vi "RMX41xx Status Check.vi"() -> ()   [LabVIEW 2023]
panel:
  out "Error Code":i32[](array[numeric])
  out "error out":errorcluster
  out "Voltage Output":dbl
  out "Current Output":dbl
  in  "Wait Before Query (1550 ms)":u32=1550
  in  "Output Current (0 A)":dbl
  in  "Output Voltage (0 V)":dbl
  in  "Operation Mode (0: Constant Current)":i32(ring) items=["Constant Current", "Constant Voltage"]
  out "error out 2":errorcluster
  out "Error":bool
  out "Status":i32
  out "resulting string":string
  in  "VISA resource name":refnum<visa-resource-name>="TCPIP0::169.254.100.192::inst0::INSTR"
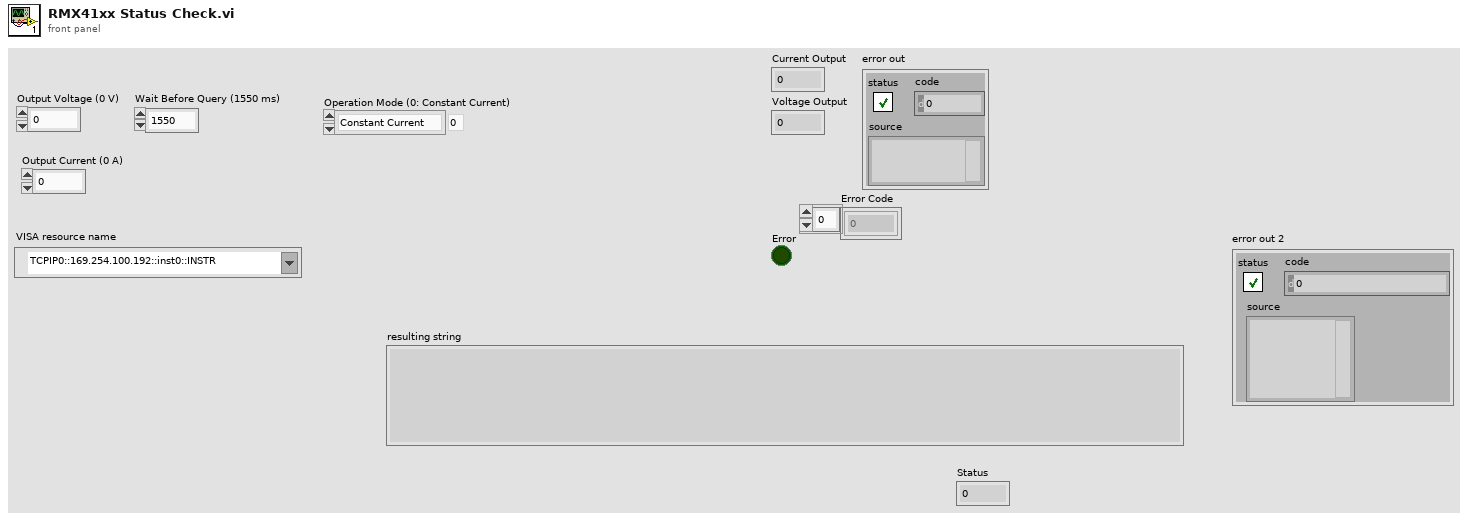
[diagram p1: front panel]
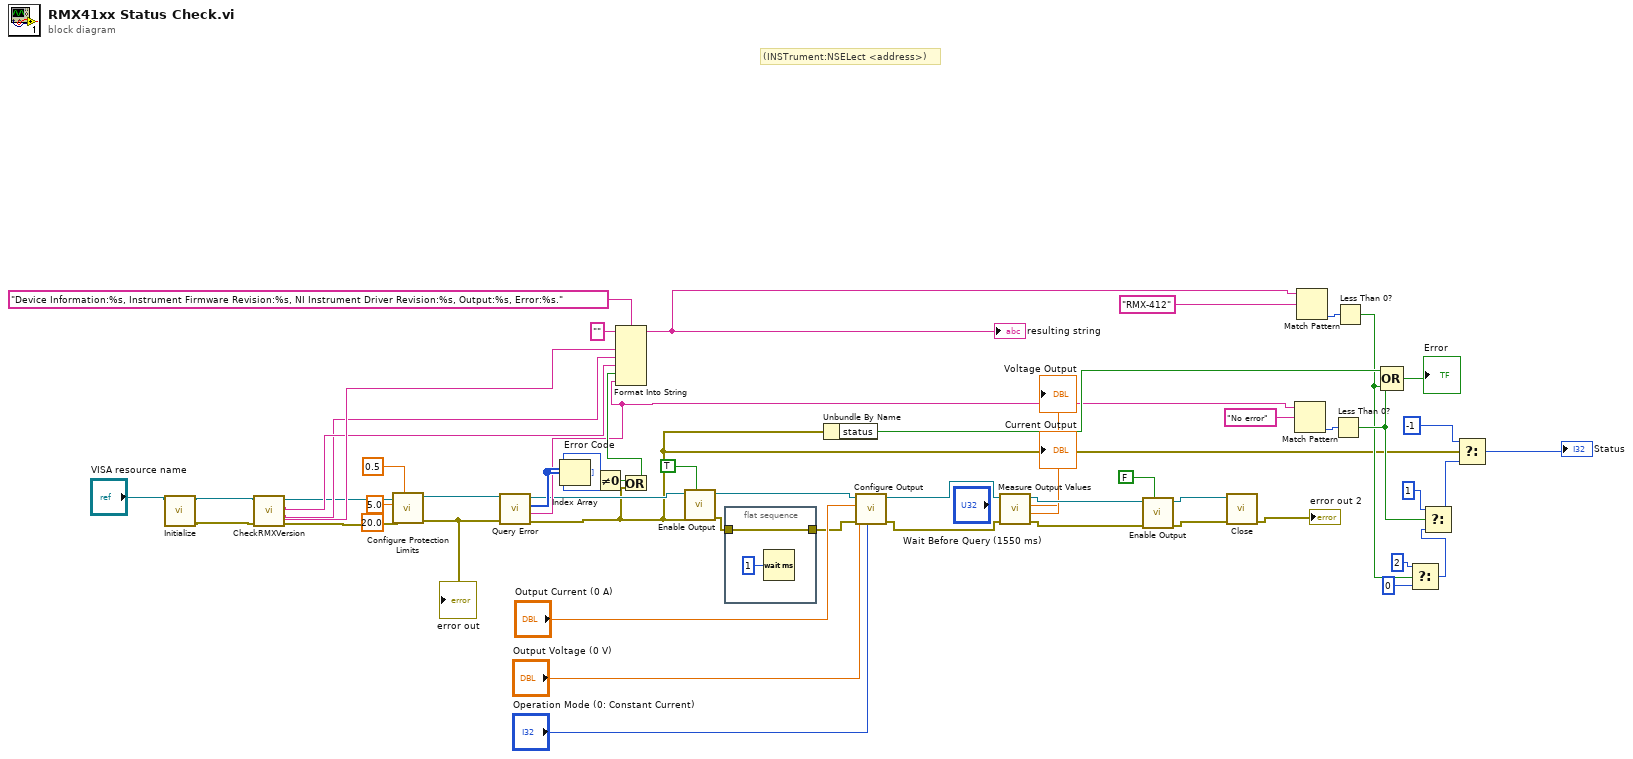
[diagram p0: block diagram]
diagram:
  # "(INSTrument:NSELect <address>)"
  n1 = call "Initialize.vi"("VISA resource name"="VISA resource name") -> ("error out"=w29:errorcluster, "VISA resource name out"=w30:refnum<visa-resource-name>)  [unwired: 9 in]
  n2 = call "CheckRMXVersion.vi"("error in (no error)"=w29, "VISA resource name"=w30) -> ("error out"=w5:errorcluster, "Instrument Driver Revision"=w51:string, "Instrument Firmware Revision"=w52:string, "VISA resource name out"=w7:refnum<visa-resource-name>, "RMXInformation"=w53:string)  [unwired: 5 in]
  n3 = call "Configure Protection Limits.vi"("Over Current Protection Detection Time (0 S)"=0.5, "error in (no error)"=w5, "Overvoltage Protection Limit (0)"=20.0, "Overcurrent Protection Limit (0)"=5.0, "VISA resource name"=w7) -> ("error out"=w4:errorcluster, "VISA resource name out"=w6:refnum<visa-resource-name>)  [unwired: 5 in]
  "error out" <- w4
  n4 = call "Query Error.vi"("error in (no error)"=w4, "VISA resource name"=w6) -> ("error out"=w13:errorcluster, "Error Message"=w27:string, "Error Code"=w28:i32[], "VISA resource name out"=w14:refnum<visa-resource-name>)  [unwired: 6 in]
  "Error Code" <- w28
  n5 = Index Array(array=w28) -> (element=w33:i32)  [unwired: 1 in]
  n6 = Not Equal To 0?(x=w33) -> (x != 0?=w32:bool)
  n7 = Or(x=w32, y=w13) -> (x .or. y?=w54:bool)
  n8 = Format Into String(format string="Device Information:%s, Instrument Firmware Revision:%s, NI Instrument Driver Revision:%s, Output:%s, Error:%s.", initial string="", w53, w51, w52, w54, w27) -> (resulting string=w41:string)  [unwired: 1 in, 1 out]
  "resulting string" <- w41
  n9 = call "Enable Output.vi"("Enable Output (F: Disable)"=TRUE, "error in (no error)"=w13, "VISA resource name"=w14) -> ("error out"=w9:errorcluster, "VISA resource name out"=w12:refnum<visa-resource-name>)  [unwired: 7 in]
  n10 = flat-sequence {
    tunnel: w9 -> [w56]
    tunnel: [w56] -> w8
    frame #0 {
      n11 = Wait (ms)(milliseconds to wait=u32 1) -> ()  [unwired: 1 out]
    }
  }
  n12 = Unbundle By Name(w13) -> ("status"=w47:bool)
  n13 = call "Configure Output.vi"("Operation Mode (0: Constant Current)"="Operation Mode (0: Constant Current)", "error in (no error)"=w8, "Output Voltage (0 V)"="Output Voltage (0 V)", "Output Current (0 A)"="Output Current (0 A)", "VISA resource name"=w12) -> ("error out"=w11:errorcluster, "VISA resource name out"=w10:refnum<visa-resource-name>)  [unwired: 5 in]
  n14 = call "Measure Output Values.vi"("error in (no error)"=w11, "VISA resource name"=w10) -> ("error out"=w24:errorcluster, "Current Output"=→"Current Output":dbl, "Voltage Output"=→"Voltage Output":dbl, "VISA resource name out"=w25:refnum<visa-resource-name>)  [unwired: 6 in]
  n15 = call "Enable Output.vi"("Enable Output (F: Disable)"=FALSE, "error in (no error)"=w24, "VISA resource name"=w25) -> ("error out"=w22:errorcluster, "VISA resource name out"=w23:refnum<visa-resource-name>)  [unwired: 7 in]
  n16 = call "Close.vi"("error in (no error)"=w22, "VISA resource name"=w23) -> ("error out"=→"error out 2":errorcluster)  [unwired: 9 in]
  n17 = Match Pattern(string=w27, regular expression="No error" ("search string")) -> (offset past match=w44:i32)  [unwired: 1 in, 3 out]
  n18 = Match Pattern(string=w41, regular expression="RMX-412" ("search string")) -> (offset past match=w42:i32)  [unwired: 1 in, 3 out]
  n19 = Less Than 0?(x=w44) -> (x < 0?=w39:bool)
  n20 = Less Than 0?(x=w42) -> (x < 0?=w37:bool)
  n21 = Compound Arithmetic op=OR(w47, w39, w37) -> (→"Error":bool)
  n22 = Select(t=2 ("Status"), s=w37, f=0) -> (s? t:f=w36:i32)
  n23 = Select(t=1 ("Status"), s=w39, f=w36) -> (s? t:f=w38:i32)
  n24 = Select(t=-1 ("Status"), s=w13, f=w38) -> (s? t:f=→"Status":i32)
